vi "Выделение чисел.vi"(1 "Строка":string) -> (0 "Массив данных двойной точности":dbl[](array[numeric]) format="%.2f")   [LabVIEW 2017]
doc: "This VI is a subVI to an exercise in the LabVIEW Basics I course.\n\nFinds all numbers in the given string and puts them into an array as double-precision numbers. All of the following formats are recognized:\n123 1.23 1.23e2 1.23E2\nNo spaces or other characters may appear within the number, but any characters may appear before or after the number."
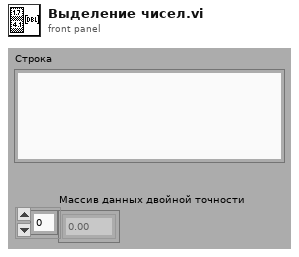
[diagram p1: front panel]
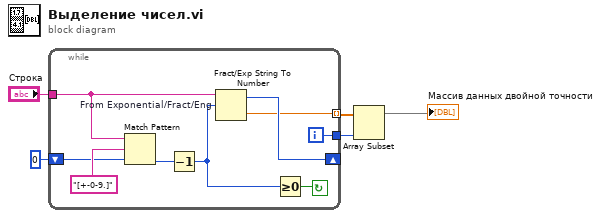
[diagram p0: block diagram]
diagram:
  n1 = while {
    tunnel: "Строка" -> [w7]
    tunnel: [w8] -> w3
    tunnel: [w9] -> w4 mode=indexing
    shift-left: 0 -> [w13]
    shift-right: [w10] -> _
    i -> [w8]
    stop <- w6 continue-if-true
    n2 = Match Pattern(string=w7, regular expression="[+-0-9.]", offset (0)=w13) -> (offset past match=w12:i32)  [unwired: 3 out]
    n3 = Decrement(x=w12) -> (x-1=w11:i32)
    n4 = Fract/Exp String To Number "From Exponential/Fract/Eng"(string=w7, offset=w11) -> (offset past number=w10:i32, number=w9:dbl)  [unwired: 2 in]
    n5 = Greater Or Equal To 0?(x=w11) -> (x >= 0?=w6:bool)
  }
  n6 = Array Subset "Array Subset"(array=w4, length=w3) -> (→"Массив данных двойной точности":dbl[])  [unwired: 1 in]
